vi "InsertData.vi"(8 "error in (no error)":errorcluster, 10 "Data Cluster":variant, 11 "object in":refnum<class "TableLogger_CSV_Actor.lvclass">) -> (0 "error out":errorcluster, 3 "object out":refnum<class "TableLogger_CSV_Actor.lvclass">)   [LabVIEW 2014, in "TableLogger_CSV_Actor.lvlib" / "TableLogger_CSV_Actor.lvclass"]
uses:
  TableLogger_CSV_Actor.lvclass
  TableLogger_CSV_Actor.lvclass/TableLogger_CSV_Actor.ctl
  TableLogger_Actor/TableLogger_Actor/TableLogger_Actor.lvclass
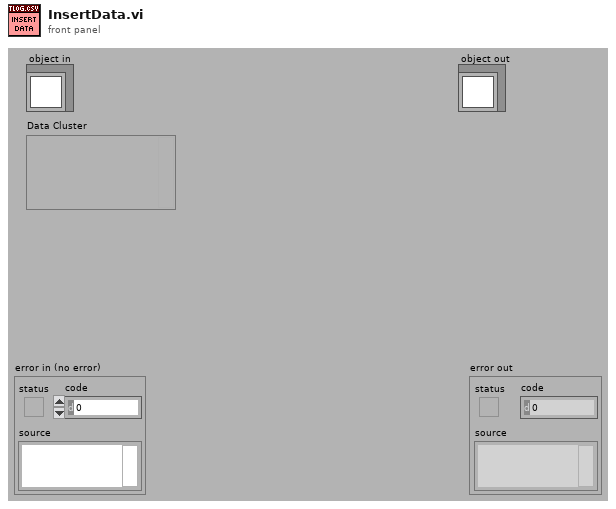
[diagram p1: front panel]
types:
  T1 = typedef "Type Descriptor Enumeration__ogtk.ctl" = enum8{"<Null>", "I8", "I16", "I32", "I64", "U8", "U16", "U32", "U64", "SGL", "DBL", "EXT", "CSG", "CDB", "CXT", "0x0F", "0x10", "0x11", "0x12", "0x13", "0x14", "Enum U8", "Enum U16", "Enum U32", "Enum U64", "SGL PQ", "DBL PQ", "EXT PQ", "CSG PQ", "CDB PQ", "CXT PQ", "0x1F", "0x20", "Boolean", "0x22", "0x23", "0x24", "0x25", "0x26", "0x27", "0x28", "0x29", "0x2A", "0x2B", "0x2C", "0x2D", "0x2E", "0x2F", "String", "0x31", "Path", "Pict", "0x34", "0x35", "0x36", "DAQ", "0x38", "0x39", "0x3A", "0x3B", "0x3C", "0x3D", "0x3E", "0x3F", "Array", "0x41", "0x42", "0x43", "0x44", "0x45", "0x46", "0x47", "0x48", "0x49", "0x4A", "0x4B", "0x4C", "0x4D", "0x4E", "0x4F", "Cluster", "0x51", "0x52", "Variant", "Waveform", "0x55", "0x56", "0x57", "0x58", "0x59", "0x5A", "0x5B", "0x5C", "0x5D", "0x5E", "0x5F", "0x60", "0x61", "0x62", "0x63", "0x64", "0x65", "0x66", "0x67", "0x68", "0x69", "0x6A", "0x6B", "0x6C", "0x6D", "0x6E", "0x6F", "Refnum"}
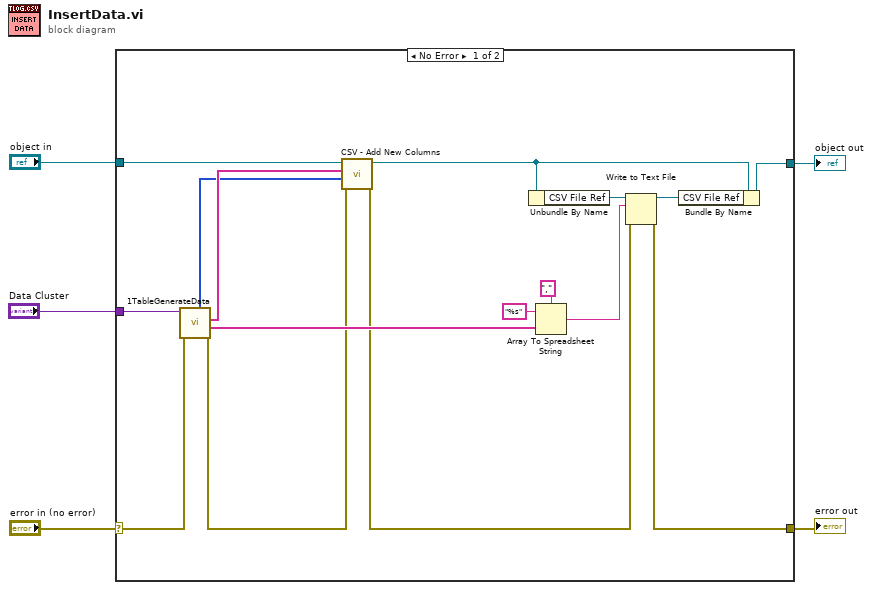
[diagram p0: block diagram]
diagram:
  n1 = case shown="No Error" "error in (no error)" {
    selector: "error in (no error)" -> [w19 w23]
    tunnel: [w18 w23] -> w4
    tunnel: [w21 w22] -> w2
    tunnel: "object in" -> [w11 w22]
    tunnel: "Data Cluster" -> [w20 _]
    frame No Error {
      n2 = call "1TableGenerateData.vi"("error in (no error)"=w19, "Cluster Variant"=w20) -> ("error out"=w9:errorcluster, "Data"=w12:string[], "Headers"=w7:string[], "LV Data Types"=w6:T1[])  [unwired: 5 in, 1 out]
      n3 = call "CSV - Add New Columns.vi"("error in (no error)"=w9, "LV Data Types"=w6, "Headers"=w7, "TableLogger_CSV_Actor in"=w11) -> ("error out"=w8:errorcluster, "TableLogger_CSV_Actor out"=w10:refnum<class "TableLogger_CSV_Actor.lvclass">)  [unwired: 6 in]
      n4 = Unbundle By Name(w10) -> ("CSV File Ref"=w17:refnum<file>)
      n5 = Array To Spreadsheet String(delimiter (Tab)=",", array=w12, 3:"%s" ("format string")) -> (spreadsheet string=w15:string)
      n6 = Write to Text File(file (use dialog)=w17, text=w15, error in=w8) -> (refnum out=w16:refnum<file>, error out=w18:errorcluster)  [unwired: 1 in, 1 out]
      n7 = Bundle By Name(cluster=w10, "CSV File Ref"=w16) -> (w21:refnum<class "TableLogger_CSV_Actor.lvclass">)
    }
    frame Error {
    }
  }
  "error out" <- w4
  "object out" <- w2
